vi "_API_BINANCE_GET_AccountAPI_BINANCETradingStatus.vi"(0 "BinanceAPI in":refnum<class "BinanceAPI_.lvclass">, 5 "Account API Trading Status":cluster{"recvWindow":i32}={"recvWindow"=5000}, 11 "error in (no error)":errorcluster) -> (4 "BinanceAPI out":refnum<class "BinanceAPI_.lvclass">, 6 "value":T1, 14 "Dane":string, 15 "error out":errorcluster)   [LabVIEW 2022 SP3, in "BinanceAPI_.lvclass"]
doc: "https://binance-docs.github.io/apidocs/spot/en/#account-api-trading-status-user_data"
uses:
  BinanceAPI_.lvclass
  BinanceAPI_.lvclass/BinanceAPI_.ctl
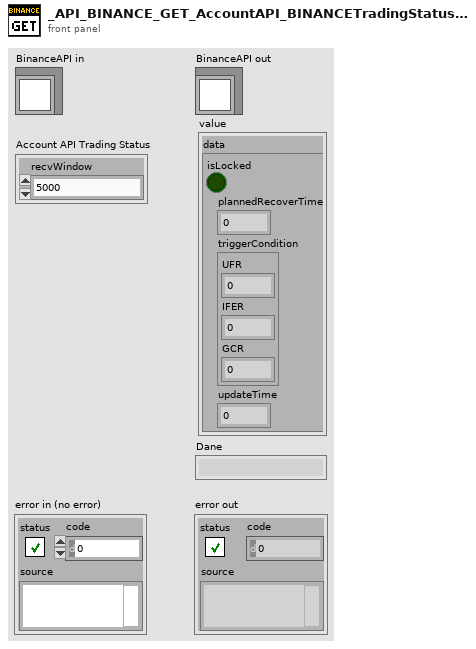
[diagram p1: front panel]
types:
  T1 = cluster{"data":cluster{"isLocked":bool, "plannedRecoverTime":dbl, "triggerCondition":cluster{"UFR":dbl, "IFER":dbl, "GCR":dbl}, "updateTime":dbl}}
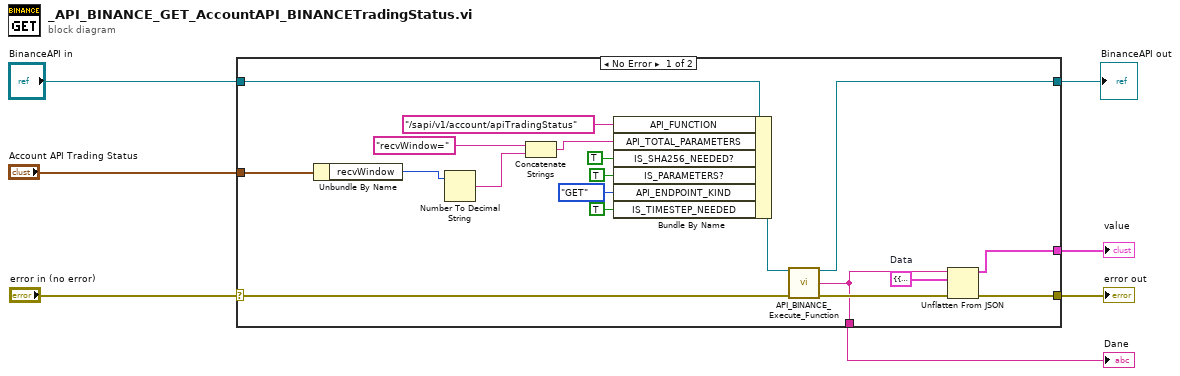
[diagram p0: block diagram]
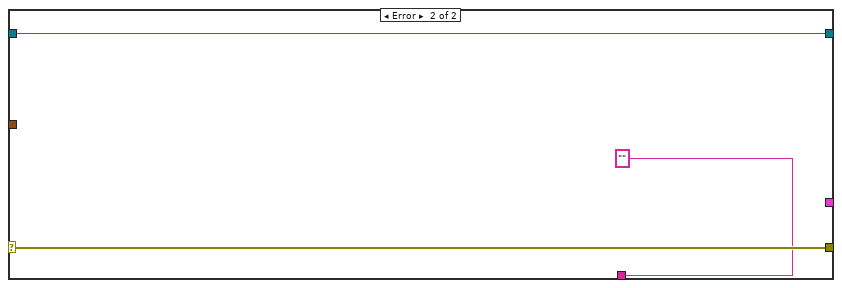
[diagram p2: hidden frame]
diagram:
  n1 = case shown="No Error" "error in (no error)" {
    selector: "error in (no error)" -> [w15 w29]
    tunnel: [w11 w29] -> w6
    tunnel: [w16 w28] -> w1
    tunnel: "BinanceAPI in" -> [w19 w28]
    tunnel: "Account API Trading Status" -> [w22 _]
    tunnel: [w10 "" ("Dane")] -> w5
    tunnel: [w8 _] -> w3
    frame No Error {
      w9 = T1 {"data"={"isLocked"=FALSE, "plannedRecoverTime"=0.0, "triggerCondition"={"UFR"=0.0, "IFER"=0.0, "GCR"=0.0}, "updateTime"=0.0}}  # Data
      n2 = Unbundle By Name(w22) -> ("recvWindow"=w13:i32)
      n3 = Number To Decimal String(number=w13) -> (decimal integer string=w12:string)  [unwired: 1 in]
      n4 = Concatenate Strings("recvWindow=" ("API_FUNCTION 2"), w12) -> (w23:string)
      n5 = Bundle By Name(cluster=w19, "API_FUNCTION"="/sapi/v1/account/apiTradingStatus", "API_TOTAL_PARAMETERS"=w23, "IS_SHA256_NEEDED?"=TRUE, "IS_PARAMETERS?"=TRUE, "API_ENDPOINT_KIND"=enum16{"POST", "DELETE", "GET", "PUT"}."GET", "IS_TIMESTEP_NEEDED"=TRUE) -> (w17:refnum<class "BinanceAPI_.lvclass">)
      n6 = call "API_BINANCE_Execute_Function.vi"("BinanceAPI in"=w17, "error in (no error)"=w15) -> ("BinanceAPI out"=w16:refnum<class "BinanceAPI_.lvclass">, "Body"=w10:string, "error out"=w14:errorcluster)  [unwired: 9 in, 2 out]
      n7 = Unflatten From JSON(JSON string=w10, type and defaults=w9, error in (no error)=w14) -> (value=w8:T1, error out=w11:errorcluster)  [unwired: 4 in]
    }
    frame Error {
    }
  }
  "error out" <- w6
  "Dane" <- w5
  "value" <- w3
  "BinanceAPI out" <- w1
